vi "To Waveform.vi"(8 "error in (no error)":errorcluster, 11 "Boolean in":refnum<class "Boolean.lvclass">) -> (0 "error out":errorcluster, 1 "Success?":bool, 3 "Waveform Array":waveform(dbl)[](array[waveform]))   [LabVIEW 2020, in "Data.lvlib" / "Boolean.lvclass"]
doc: "Interpret 'Data' as a Waveform Array. If impossible 'Success?' is set to FALSE"
uses:
  Boolean.lvclass
  Boolean.lvclass/Boolean.ctl
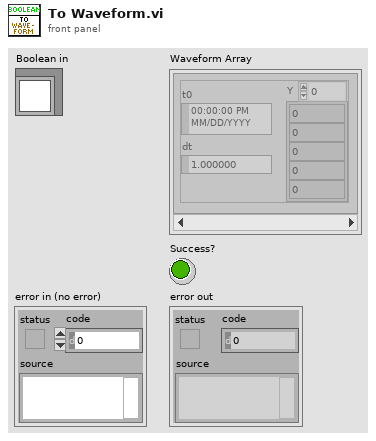
[diagram p1: front panel]
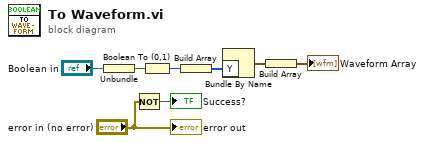
[diagram p0: block diagram]
diagram:
  n1 = Unbundle("Boolean in") -> (w7:bool)
  n2 = Not(x="error in (no error)") -> (.not. x?=→"Success?":bool)
  n3 = Boolean To (0,1)(Boolean=w7) -> (0, 1=w6:i16)
  n4 = Build Array(w6) -> (w5:i16[])
  n5 = Bundle By Name("Y"=w5) -> (w4:waveform(i16))  [unwired: 1 in]
  n6 = Build Array(w4) -> (→"Waveform Array":waveform(i16)[])
  "error out" <- "error in (no error)"
